vi "Intro_1.vi"() -> ()   [LabVIEW 2018]
panel:
  out "X/Y":dbl
  in  "Y":i8
  in  "Slide 3":dbl(slide) scale=0.0..9.0
  in  "Slide 2":dbl(slide) scale=0.0..9.0
  out "Gauge":dbl(knob) scale=0.0..9.0
  in  "Slide":dbl(slide) min=0.0 max=9.0 scale=0.0..9.0 scale format="%1d"
  in  "X":i8
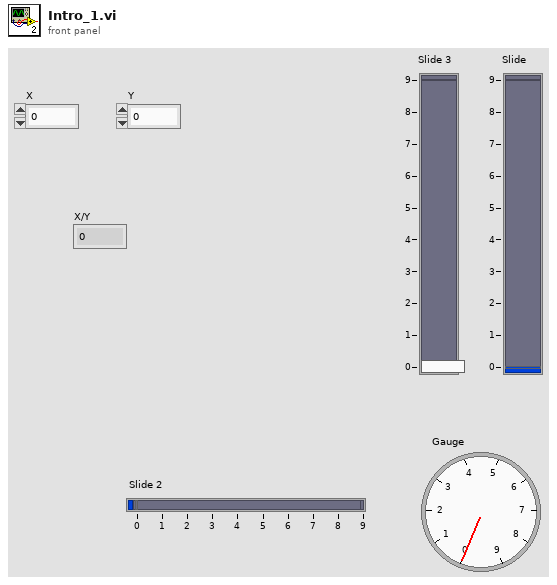
[diagram p1: front panel]
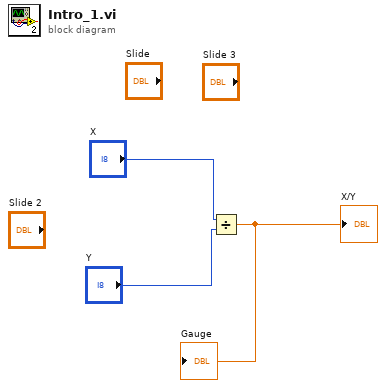
[diagram p0: block diagram]
diagram:
  n1 = Divide(x="X", y="Y") -> (x/y=→"Gauge" →"X/Y":dbl)
